vi "Read Config.vi"(8 "error in (no error)":errorcluster, 10 "Resource In":variant, 11 "Analyze Parameter Spectral Calibration in":refnum<class "Analyze Parameter Spectral Calibration.lvclass">) -> (0 "error out":errorcluster, 2 "Resource Out":variant, 3 "Analyze Parameter Spectral Calibration out":refnum<class "Analyze Parameter Spectral Calibration.lvclass">)   [LabVIEW 2020, in "Analyze Parameter Spectral Calibration.lvclass"]
uses:
  Analyze Parameter Spectral Calibration.lvclass
  C:/POLARIS Programme/POLARIS-AS-3-Cams/Submodules/HIJ Vision/Analyze/Analyze Parameter/Analyze Parameter Base/Analyze Parameter Base.lvclass
  <vilib>/Utility/config.llb/Config Data RefNum.ctl
  Analyze Parameter Spectral Calibration.lvclass/Analyze Parameter Spectral Calibration.ctl
  <vilib>/Utility/config.llb/Read Key (I32).vi
  <vilib>/Utility/config.llb/Read Key (Double).vi
  <vilib>/Utility/config.llb/NI_LVConfig.lvlib
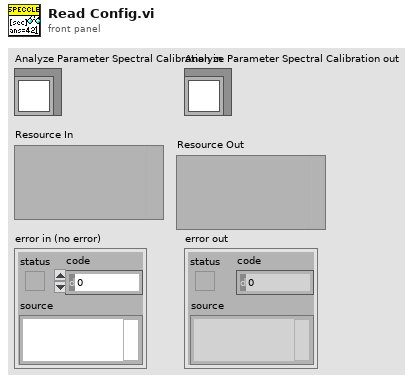
[diagram p1: front panel]
types:
  T1 = typedef "NI_LVConfig.lvlib/Config Data RefNum.ctl" = refnum<k1>
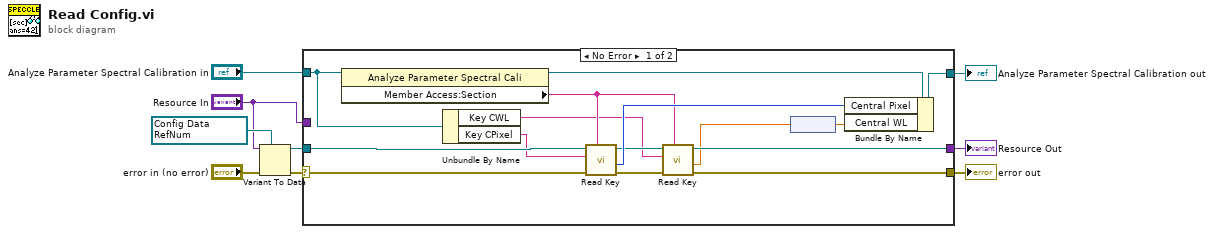
[diagram p0: block diagram]
diagram:
  w9 = T1 refnum items=["config data"] ("refnum")
  n1 = Variant To Data(error in="error in (no error)", type=w9, Variant="Resource In") -> (data=w8:T1, error out=w7:errorcluster)
  n2 = case shown="No Error" w7 {
    selector: w7 -> [w18 w26]
    tunnel: w8 -> [w24 _]
    tunnel: "Analyze Parameter Spectral Calibration in" -> [w19 w25]
    tunnel: [w22 w25] -> w3
    tunnel: [w16 w27] -> w2
    tunnel: [w14 w26] -> w1
    tunnel: "Resource In" -> [_ w27]
    frame No Error {
      n3 = property class="Analyze Parameter Spectral Cali"(reference=w19) -> (reference out=w20:refnum<class "Analyze Parameter Spectral Calibration.lvclass">, "Member Access:Section"=w13:string)  [unwired: 1 in, 1 out]
      n4 = Unbundle By Name(w19) -> ("Key CWL"=w10:string, "Key CPixel"=w21:string)
      n5 = call-poly <vilib>:"Read Key.vi"("section"=w13, "error in (no error)"=w18, "key"=w21, "refnum"=w24) -> ("error out"=w15:errorcluster, "value"=w23:i32, "refnum out"=w17:T1)  [unwired: 4 in, 1 out]
      n6 = call-poly <vilib>:"Read Key.vi"("section"=w13, "error in (no error)"=w15, "key"=w10, "refnum"=w17) -> ("error out"=w14:errorcluster, "value"=w12:dbl, "refnum out"=w16:T1)  [unwired: 4 in, 1 out]
      n7 = node(w12) -> (w11:dbl[unit])
      n8 = Bundle By Name(cluster=w20, "Central Pixel"=w23, "Central WL"=w11) -> (w22:refnum<class "Analyze Parameter Spectral Calibration.lvclass">)
    }
    frame Error {
    }
  }
  "error out" <- w1
  "Analyze Parameter Spectral Calibration out" <- w3
  "Resource Out" <- w2
